vi "Check Freq Cal Done.vi"(8 "error in (no error)":errorcluster) -> (0 "error out":errorcluster, 3 "function return":bool)   [LabVIEW 2013, in "QCAWLAN_DLL.lvlib"]
doc: "QCA_DLL_Export bool CheckFreqCalDone();"
uses:
  QCAWLAN_DLL.lvlib
  QCAWLAN_DLL.dll
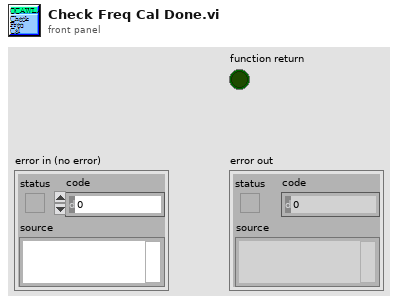
[diagram p1: front panel]
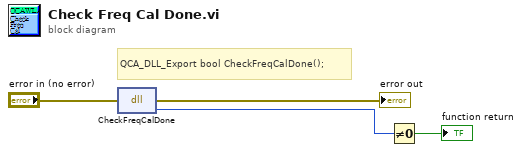
[diagram p0: block diagram]
diagram:
  # "QCA_DLL_Export bool CheckFreqCalDone();"
  n1 = dll-call lib="C:/Connectivity Client - MIMO/PlugIn/QCAWLAN_DLL.*" fn="CheckFreqCalDone"(error in="error in (no error)") -> (error out=→"error out":errorcluster, w3:u8)  [unwired: 2 in, 1 out]
  n2 = Not Equal To 0?(x=w3) -> (x != 0?=→"function return":bool)
